vi "VISA AMI430 Open.vi"(8 "error in (no error)":errorcluster, 10 "Timeout (ms)":u32=3000, 11 "VISA session":refnum<visa-resource-name>="TCPIP::146.201.232.88::7180::SOCKET") -> (0 "error out":errorcluster {"code" format="%.0x"}, 2 "Hello string":string, 3 "dup VISA Session":refnum<visa-resource-name>)   [LabVIEW 2025]
doc: "Author: Scott Hannahs <sth@magnet.fsu.edu>\n\nThis software is licensed for use under the “MIT License\"\nCopyright (c) 2025 Scott Hannahs, sth@sth@magnet.sthnet.net\n\nPermission is hereby granted, free of charge, to any person obtaining a copy of this software and associated documentation files (the \"Software\"), to deal in the Software without restriction, including without limitation the rights to use, copy, modify, merge, publish, distribute, sublicense, and/or sell copies of the Software, and to permit persons to whom the Software is furnished to do so, subject to the following conditions: The above copyright notice and this permission notice shall be included in all copies or substantial portions of the Software.\n\nTHE SOFTWARE IS PROVIDED \"AS IS\", WITHOUT WARRANTY OF ANY KIND, EXPRESS OR IMPLIED, INCLUDING BUT NOT LIMITED TO THE WARRANTIES OF MERCHANTABILITY, FITNESS FOR A PARTICULAR PURPOSE AND NONINFRINGEMENT. IN NO EVENT SHALL THE AUTHORS OR COPYRIGHT HOLDERS BE LIABLE FOR ANY CLAIM, DAMAGES OR OTHER LIABILITY, WHETHER IN AN ACTION OF CONTRACT, TORT OR OTHERWISE, ARISING FROM, OUT OF OR IN CONNECTION WITH THE SOFTWARE OR THE USE OR OTHER DEALINGS IN THE SOFTWARE."
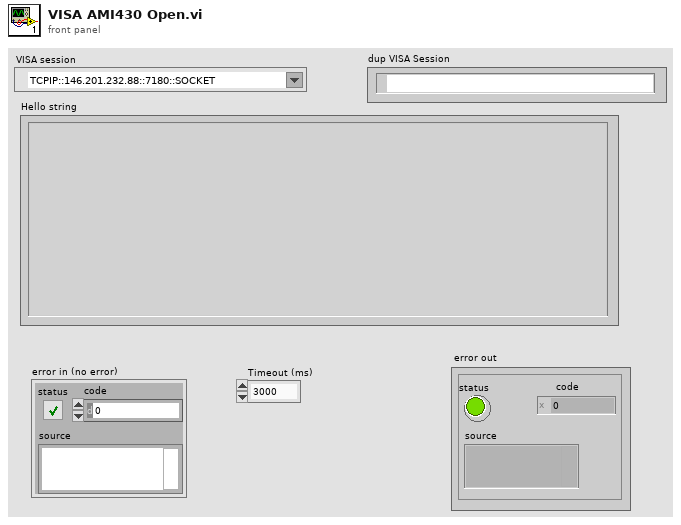
[diagram p1: front panel]
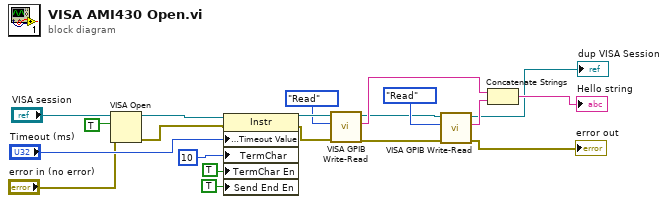
[diagram p0: block diagram]
diagram:
  n1 = VISA Open(duplicate session (F)=TRUE, error in (no error)="error in (no error)", VISA resource name="VISA session") -> (VISA resource name=w19:refnum<visa-resource-name>, error out=w17:errorcluster)  [unwired: 2 in]
  n2 = property class="Instr"(reference=w19, error in=w17, "General Settings:Timeout Value"="Timeout (ms)", "TermChar"=u8 10 ("Message Based Settings:Termination Character"), "TermChar En"=TRUE ("Message Based Settings:Termination Character Enable"), "Send End En"=TRUE ("Message Based Settings:Send End Enable")) -> (reference out=w15:refnum<visa-resource-name>, error out=w16:errorcluster)
  n3 = call "VISA GPIB Write-Read.vi"("error in (no error)"=w16, "Action"=enum16{"Write", "Read", "Write & Read"}."Read", "VISA resource name"=w15) -> ("error out"=w2:errorcluster, "String Returned"=w8:string, "dup VISA Session"=w5:refnum<visa-resource-name>)  [unwired: 5 in, 1 out]
  n4 = call "VISA GPIB Write-Read.vi"("error in (no error)"=w2, "Action"=enum16{"Write", "Read", "Write & Read"}."Read", "VISA resource name"=w5) -> ("error out"=→"error out":errorcluster, "String Returned"=w7:string, "dup VISA Session"=→"dup VISA Session":refnum<visa-resource-name>)  [unwired: 5 in, 1 out]
  n5 = Concatenate Strings(w8, w7) -> (→"Hello string":string)
